vi "Delete Buffer.vi"(11 "BufferWrites1SamDBL in":refnum<class "BufferWrites1SamDBL.lvclass">) -> (3 "BufferWrites1SamDBL out":refnum<class "BufferWrites1SamDBL.lvclass">)   [LabVIEW 2023, in "BufferWrites1SamDBL.lvclass"]
uses:
  BufferWrites1SamDBL.lvclass
  BufferWrites1SamDBL.lvclass/BufferWrites1SamDBL.ctl
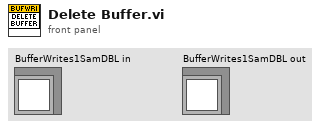
[diagram p1: front panel]
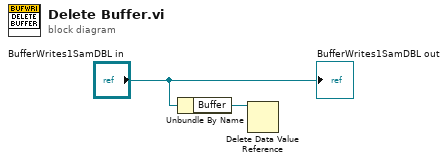
[diagram p0: block diagram]
diagram:
  n1 = Unbundle By Name("BufferWrites1SamDBL in") -> ("Buffer"=w1:refnum<data-value>)
  n2 = Delete Data Value Reference(data value reference=w1) -> ()  [unwired: 1 in, 2 out]
  "BufferWrites1SamDBL out" <- "BufferWrites1SamDBL in"
